vi "Callback Change Physical Channel.vi"(6 "Variant":variant, 8 "error in (no error)":errorcluster, 9 "Old Values":string[][](array[string]), 10 "object ref in":T1, 11 "Table Change":T2) -> (0 "error out":errorcluster)   [LabVIEW 2014, in "Daqmx Module editor node.lvclass"]
doc: "This VI gets called automatically when changes are made to the 'Name' column of the table and must handle changes appropriately. Register this callback using the appropriate 'Define Column' VI from the Table API."
uses:
  Daqmx Module editor node.lvclass
  <vilib>/NI/DCAF/Tag Editor Core/Table API/Table Manager/Cell Change.ctl
  <vilib>/NI/DCAF/Tag Editor Core/Table API/Table Manager/object ref.ctl
  <vilib>/NI/DCAF/Tag Editor Core/Configuration Editor/Classes/Engine Parent/Engine Parent Editor Node.lvclass
  <vilib>/NI/DCAF/Tag Editor Core/Configuration Editor/Classes/Module editor node/module editor node.lvclass
  module/configuration/Daqmx Module configuration.lvclass
  module/configuration/Daqmx Module configuration.lvclass/Daqmx Module configuration.ctl
  module/configuration/Get Line Name.vi
  <vilib>/NI/Tag Bus Module Framework/module configuration/FindDuplicate.vi
  <vilib>/Utility/error.llb/Error Cluster From Error Code.vi
  <vilib>/NI/Tag Bus Module Framework/channel/TBM channel.lvclass
  <vilib>/NI/DCAF/Tag Editor Core/Table API/Table Manager.lvlib
  <vilib>/NI/DCAF/Tag Editor Core/Table API/Table Manager/Table Manager.lvclass
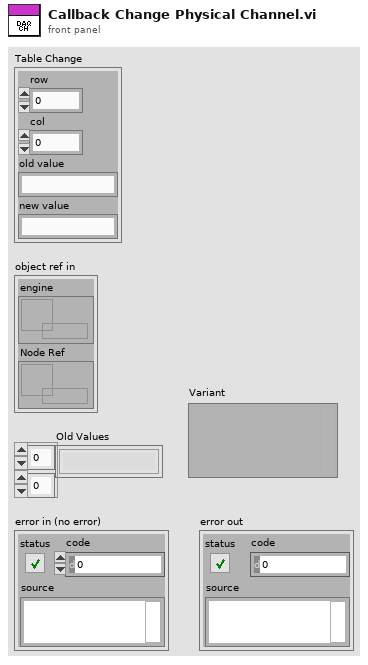
[diagram p1: front panel]
types:
  T1 = typedef "Table Manager.lvlib/Table Manager.lvclass/object ref.ctl" = cluster{"engine":refnum<data-value>, "Node Ref":refnum<data-value>}
  T2 = typedef "Table Manager.lvlib/Cell Change.ctl" = cluster{"row":i32, "col":i32, "old value":string, "new value":string}
  T3 = typedef "Daqmx Module configuration.lvclass/Line.ctl" = cluster{"channel":refnum<class "TBM channel.lvclass">, "Physical Channel":string, "Channel Type":T4, "Parameters":variant}
  T4 = typedef "Daqmx Module configuration.lvclass/Channel Type.ctl" = enum16{"Analog", "Digital"}
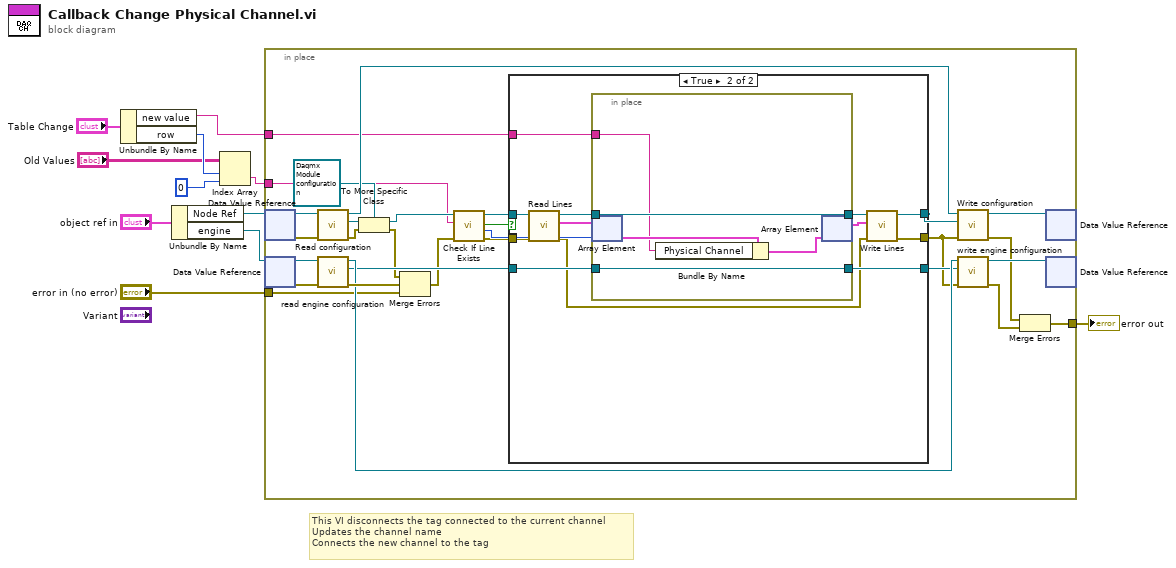
[diagram p0: block diagram]
diagram:
  # "This VI disconnects the tag connected to the current channel\nUpdates the channel name\nConnects the new channel to the tag"
  n1 = Unbundle By Name("Table Change") -> ("new value"=w5:string, "row"=w3:i32)
  n2 = Unbundle By Name("object ref in") -> ("Node Ref"=w8:refnum<data-value>, "engine"=w7:refnum<data-value>)
  n3 = Index Array(array="Old Values", index (row)=w3, index (col)=0 ("disabled index (col)")) -> (element=w1:string)
  n4 = in-place {
    in-place-border: [w32] -> w11
    in-place-border: "error in (no error)" -> [w28]
    in-place-border: w5 -> [w24]
    in-place-border: w1 -> [w12]
    n5 = in-place-dvr #1(w8) -> (w22:refnum<class "module editor node.lvclass">, w31:errorcluster)
    n6 = in-place-dvr #2(w7) -> (w39:refnum<class "Engine Parent Editor Node.lvclass">, w40:errorcluster)
    n7 = call-dynamic "Read configuration.vi"("error in"=w31, "NISE_CEF_serializable node in"=w22) -> ("error out"=w14:errorcluster, "configuration"=w29:refnum<class "NISE_CEF_serializable configuration.lvclass">, "NISE_CEF_serializable node out"=w30:refnum<class "module editor node.lvclass">)  [unwired: 7 in]
    n8 = call <vilib>:"read engine configuration.vi"("error in"=w40, "Engine Parent Editor Node in"=w39) -> ("error out"=w36:errorcluster, "engine configuration"=w19:refnum<class "engine configuration.lvclass">, "Engine Parent Editor Node out"=w35:refnum<class "Engine Parent Editor Node.lvclass">)  [unwired: 7 in]
    n9 = To More Specific Class(target class=refnum<class "Daqmx Module configuration.lvclass"> refnum ("tag bus configurable plugin module configuration"), reference=w29, error in=w14) -> (specific class reference=w21:refnum<class "Daqmx Module configuration.lvclass">, error out=w13:errorcluster)
    n10 = Merge Errors(w13, w36, w28) -> (w17:errorcluster)
    n11 = call-dynamic "Check If Line Exists.vi"("error in"=w17, "Name to Locate"=w12, "Daqmx Module configuration in"=w21) -> ("error out"=w18:errorcluster, "Index"=w25:i32, "Daqmx Module configuration out"=w16:refnum<class "Daqmx Module configuration.lvclass">, "Found?"=w23:bool)  [unwired: 4 in, 1 out]
    n12 = case shown="True" w23 {
      tunnel: [w43 w56] -> w26
      tunnel: w16 -> [w43 w55]
      tunnel: w25 -> [_ w52]
      tunnel: w24 -> [_ w51]
      tunnel: w19 -> [w42 w50]
      tunnel: [w42 w49] -> w20
      tunnel: [w41 w48] -> w15
      tunnel: w18 -> [w41 w45]
      frame False {
      }
      frame True {
        n13 = call "Read Lines.vi"("error in (no error)"=w45, "Daqmx Module configuration in"=w55) -> ("error out"=w44:errorcluster, "Lines"=w54:T3[], "Daqmx Module configuration out"=w47:refnum<class "Daqmx Module configuration.lvclass">)  [unwired: 7 in]
        n14 = in-place {
          in-place-border: w51 -> [w57]
          in-place-border: w50 -> [w61]
          in-place-border: [w61] -> w49
          in-place-border: w47 -> [w60]
          in-place-border: [w60] -> w46
          n15 = in-place-array #3(w54, w52) -> (w59:T3)
          n16 = Bundle By Name(cluster=w59, "Physical Channel"=w57) -> (w58:T3)
          n17 = in-place-array #3(w58) -> (w53:T3[])  [unwired: 1 out]
        }
        n18 = call "Write Lines.vi"("error in (no error)"=w44, "Lines"=w53, "Daqmx Module configuration in"=w46) -> ("error out"=w48:errorcluster, "Daqmx Module configuration out"=w56:refnum<class "Daqmx Module configuration.lvclass">)  [unwired: 7 in]
      }
    }
    n19 = call-dynamic "Write configuration.vi"("error in"=w15, "configuration"=w26, "NISE_CEF_serializable node in"=w30) -> ("error out"=w33:errorcluster, "NISE_CEF_serializable node out"=w37:refnum<class "module editor node.lvclass">)  [unwired: 7 in]
    n20 = call <vilib>:"write engine configuration.vi"("error in"=w15, "engine configuration"=w20, "Engine Parent Editor Node in"=w35) -> ("error out"=w34:errorcluster, "Engine Parent Editor Node out"=w38:refnum<class "Engine Parent Editor Node.lvclass">)  [unwired: 7 in]
    n21 = Merge Errors(w33, w34) -> (w32:errorcluster)
    n22 = in-place-dvr #1(w37) -> ()  [unwired: 2 out]
    n23 = in-place-dvr #2(w38) -> ()  [unwired: 2 out]
  }
  "error out" <- w11
